vi "GetScanDelay.vi"(8 "Error In":errorcluster, 11 "Keithley 7001 In":refnum<visa-resource-name>) -> (0 "Error Out":errorcluster, 2 "Delay (sec)":dbl, 3 "Keithley 7001 Out":refnum<visa-resource-name>)   [LabVIEW 2012, in "Keithley-7001.lvlib"]
uses:
  Keithley-7001.lvlib
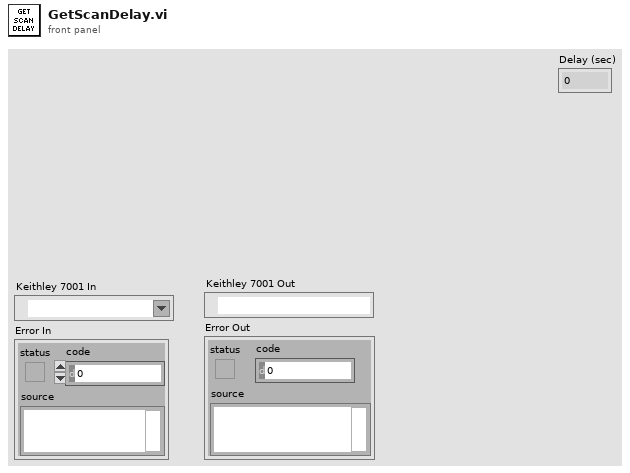
[diagram p1: front panel]
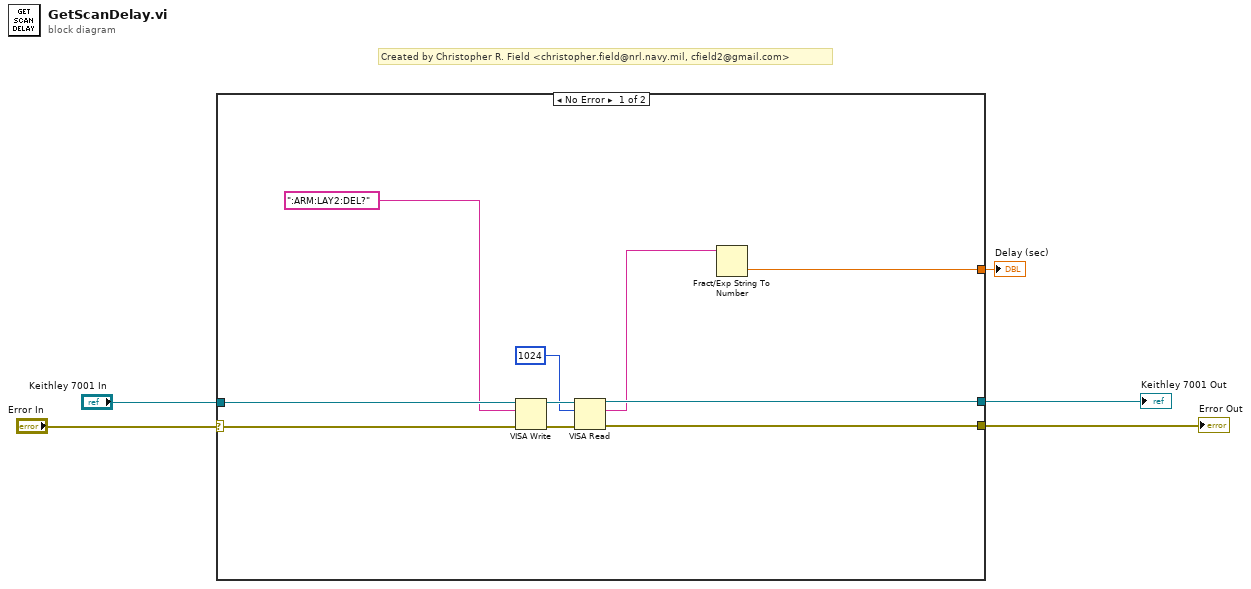
[diagram p0: block diagram]
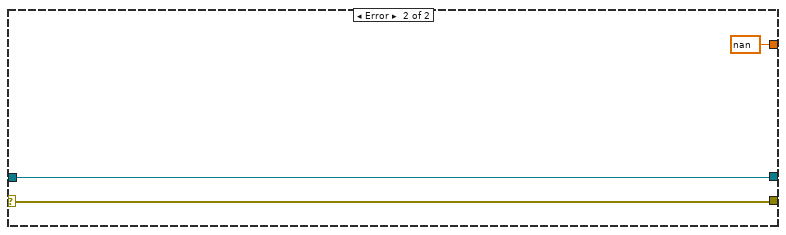
[diagram p2: hidden frame]
diagram:
  # "Created by Christopher R. Field <christopher.field@nrl.navy.mil, cfield2@gmail.com>"
  n1 = case shown="No Error" "Error In" {
    selector: "Error In" -> [w8 w17]
    tunnel: "Keithley 7001 In" -> [w13 w18]
    tunnel: [w12 w18] -> w4
    tunnel: [w11 w17] -> w3
    tunnel: [w6 nan] -> w1
    frame No Error {
      n2 = VISA Write(VISA resource name=w13, write buffer=":ARM:LAY2:DEL?", error in (no error)=w8) -> (VISA resource name out=w15:refnum<visa-resource-name>, error out=w14:errorcluster)  [unwired: 1 out]
      n3 = VISA Read(VISA resource name=w15, byte count=u32 1024, error in (no error)=w14) -> (VISA resource name out=w12:refnum<visa-resource-name>, read buffer=w7:string, error out=w11:errorcluster)  [unwired: 1 out]
      n4 = Fract/Exp String To Number(string=w7) -> (number=w6:dbl)  [unwired: 3 in, 1 out]
    }
    frame Error {
    }
  }
  "Keithley 7001 Out" <- w4
  "Error Out" <- w3
  "Delay (sec)" <- w1
